vi "SerrurreV2.vi"() -> ()   [LabVIEW 2018]
uses:
  Global 5.vi
panel:
  in  "stop":bool
  out "2D Picture":picture
  out "Numeric 3":u32
  out "Numeric 2":u32
  out "Numeric":dbl
  out "Boolean 2":bool
  out "Boolean":bool
  in  "OK Button":bool
  in  "Dial 3":i8(knob) min=0 max=9 scale=0.0..9.0
  in  "Dial 2":i8(knob) min=0 max=9 scale=0.0..9.0
  in  "Dial":i8(knob)=1 min=0 max=9 scale=0.0..9.0
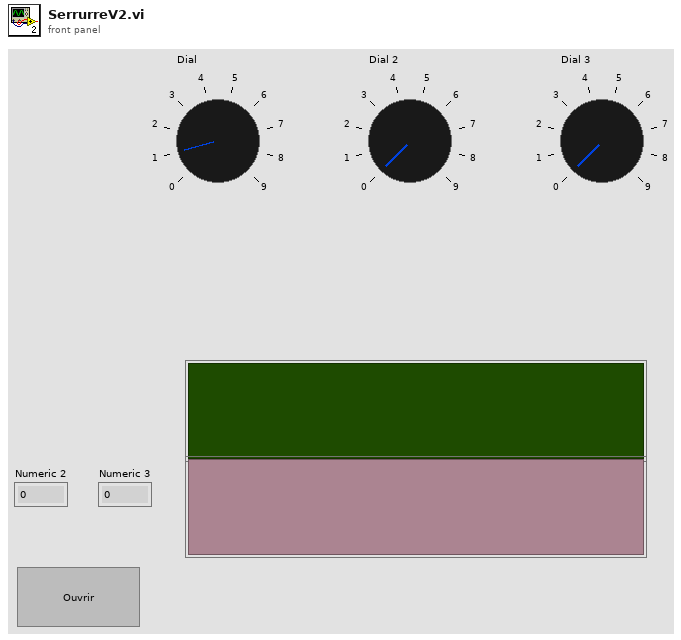
[diagram p1: front panel]
types:
  T1 = typedef "imagedata.ctl" = cluster{"image type":i32, "image depth":i32, "image":u8[], "mask":u8[], "colors":u32[], "Rectangle":cluster{"left":i16, "top":i16, "right":i16, "bottom":i16}}
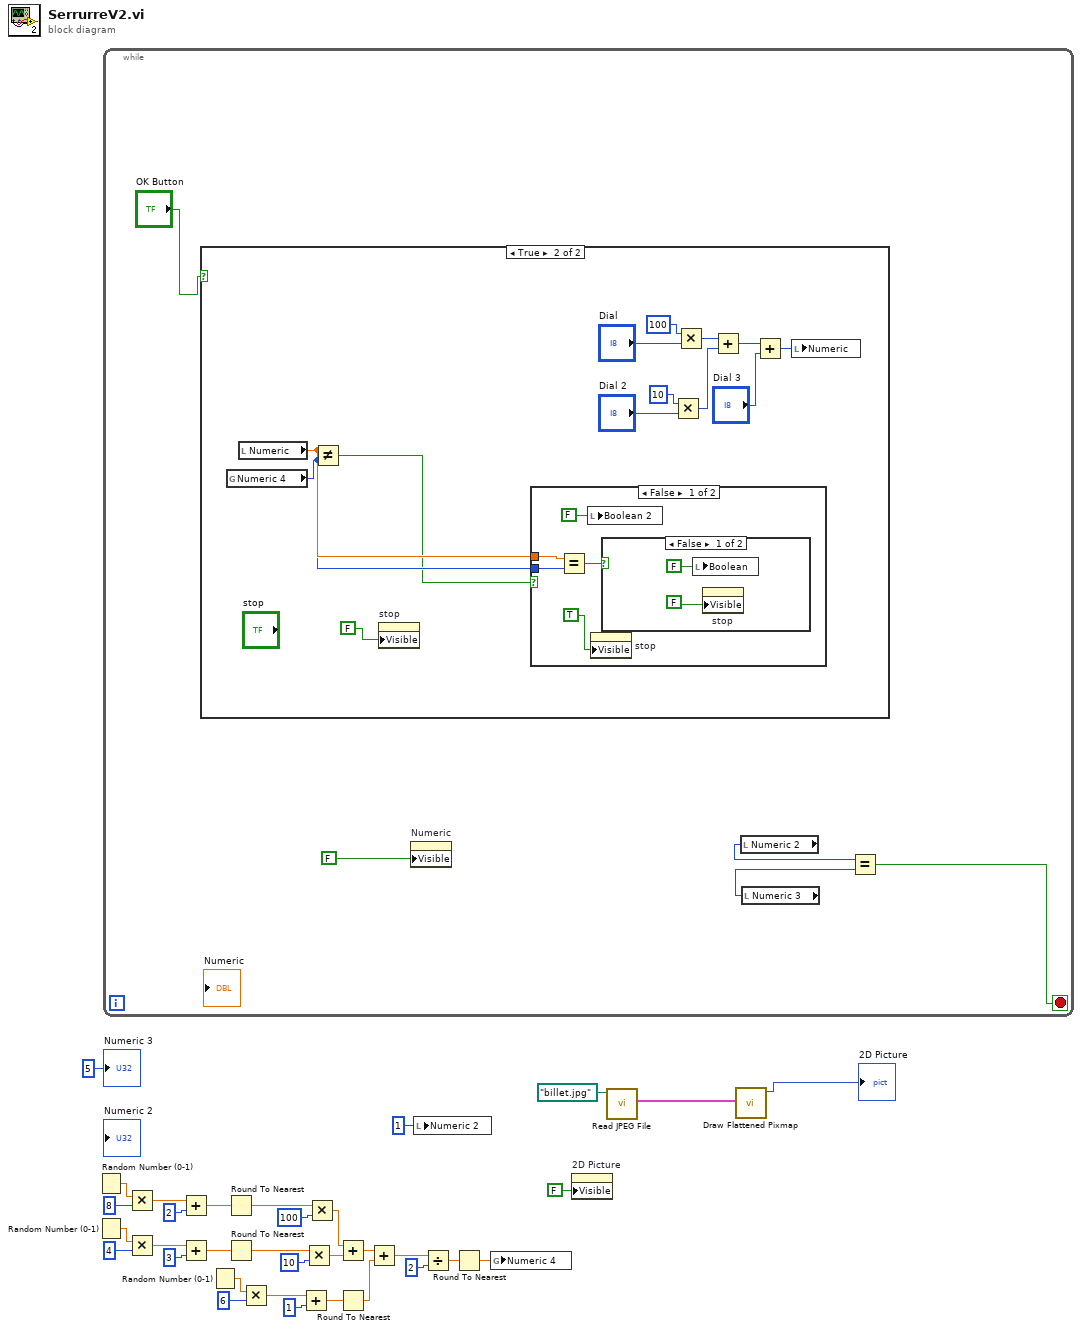
[diagram p0: block diagram]
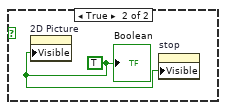
[diagram p3: hidden frame]
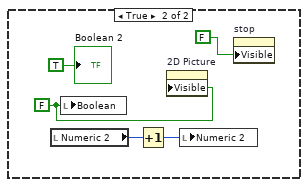
[diagram p4: hidden frame]
diagram:
  n1 = Random Number (0-1)() -> (number: 0 to 1=w33:dbl)
  n2 = Random Number (0-1)() -> (number: 0 to 1=w28:dbl)
  n3 = while {
    stop <- w37 stop-if-true
    n4 = case shown="True" "OK Button" {
      frame False {
      }
      frame True {
        n5 = global read "Global 5.vi" "Numeric 4"() -> (w50:u32)
        n6 = local read "Numeric"() -> (w51:dbl)
        n7 = Not Equal?(x=w51, y=w50) -> (x != y?=w49:bool)
        n8 = property on="stop" class="Bool"("Visible"=FALSE) -> ()  [unwired: 2 in, 2 out]
        n9 = case shown="False" w49 {
          tunnel: w50 -> [w55 _]
          tunnel: w51 -> [w54 _]
          frame False {
            n10 = Equal?(x=w54, y=w55) -> (x = y?=w56:bool)
            n11 = local write "Boolean 2"(FALSE ("Boolean 2")) -> ()
            n12 = property on="stop" class="Bool"("Visible"=TRUE) -> ()  [unwired: 2 in, 2 out]
            n13 = case shown="False" w56 {
              frame False {
                n14 = local write "Boolean"(FALSE ("Boolean")) -> ()
                n15 = property on="stop" class="Bool"("Visible"=FALSE) -> ()  [unwired: 2 in, 2 out]
              }
              frame True {
                w59 = TRUE ("Boolean")
                n16 = property on="2D Picture" class="Pict"("Visible"=w59) -> ()  [unwired: 2 in, 2 out]
                n17 = property on="stop" class="Bool"("Visible"=w59) -> ()  [unwired: 2 in, 2 out]
                "Boolean" <- w59
              }
            }
          }
          frame True {
            w61 = FALSE ("Boolean")
            n18 = local read "Numeric 2"() -> (w62:u32)
            n19 = local write "Boolean"(w61) -> ()
            n20 = Increment(x=w62) -> (x+1=w63:u32)
            n21 = property on="2D Picture" class="Pict"("Visible"=w61) -> ()  [unwired: 2 in, 2 out]
            n22 = local write "Numeric 2"(w63) -> ()
            n23 = property on="stop" class="Bool"("Visible"=FALSE) -> ()  [unwired: 2 in, 2 out]
            "Boolean 2" <- TRUE ("Boolean 2")
          }
        }
        n24 = Multiply(x=10, y="Dial 2") -> (x*y=w45:i32)
        n25 = Multiply(x=100, y="Dial") -> (x*y=w46:i32)
        n26 = Add(x=w46, y=w45) -> (x+y=w43:i32)
        n27 = Add(x=w43, y="Dial 3") -> (x+y=w42:i32)
        n28 = local write "Numeric"(w42) -> ()
      }
    }
    n29 = property on="Numeric" class="DigNum (strict)"("Visible"=FALSE) -> ()  [unwired: 2 in, 2 out]
    n30 = local read "Numeric 2"() -> (w35:u32)
    n31 = local read "Numeric 3"() -> (w36:u32)
    n32 = Equal?(x=w35, y=w36) -> (x = y?=w37:bool)
  }
  n33 = Multiply(x=w33, y=8) -> (x*y=w32:dbl)
  n34 = Multiply(x=w28, y=4) -> (x*y=w27:dbl)
  n35 = Add(x=w32, y=2) -> (x+y=w31:dbl)
  n36 = Add(x=w27, y=3) -> (x+y=w26:dbl)
  n37 = Random Number (0-1)() -> (number: 0 to 1=w23:dbl)
  n38 = Round To Nearest(number=w31) -> (nearest integer value=w16:dbl)
  n39 = Round To Nearest(number=w26) -> (nearest integer value=w15:dbl)
  n40 = Multiply(x=w23, y=6) -> (x*y=w22:dbl)
  n41 = Add(x=w22, y=1) -> (x+y=w21:dbl)
  n42 = Multiply(x=w15, y=10) -> (x*y=w13:dbl)
  n43 = Multiply(x=w16, y=100) -> (x*y=w14:dbl)
  n44 = Add(x=w14, y=w13) -> (x+y=w18:dbl)
  n45 = Round To Nearest(number=w21) -> (nearest integer value=w17:dbl)
  n46 = Add(x=w18, y=w17) -> (x+y=w10:dbl)
  n47 = local write "Numeric 2"(u32 1 ("Numeric 2")) -> ()
  n48 = Divide(x=w10, y=2) -> (x/y=w8:dbl)
  n49 = Round To Nearest(number=w8) -> (nearest integer value=w7:dbl)
  n50 = global write "Global 5.vi" "Numeric 4"(w7) -> ()
  n51 = property on="2D Picture" class="Pict"("Visible"=FALSE) -> ()  [unwired: 2 in, 2 out]
  n52 = call <vilib>:"Read JPEG File.vi"("path to JPEG file"=path "billet.jpg") -> ("image data"=w3:T1)  [unwired: 8 in, 2 out]
  n53 = call <vilib>:"Draw Flattened Pixmap.vi"("image data"=w3) -> ("new picture"=→"2D Picture":picture)  [unwired: 8 in]
  "Numeric 3" <- u32 5 ("Numeric 3")
